vi "Read Response.vi"(8 "error in":errorcluster, 11 "Axis in":refnum<class "Axis.lvclass">) -> (0 "error out":errorcluster, 2 "Success?":bool, 3 "Axis out":refnum<class "Axis.lvclass">)   [LabVIEW 2018, in "Axis.lvlib" / "Axis.lvclass"]
doc: "This VI is used in conjunction with Send Command. Send Command, when using certain types, will send a command to the instrument. Read Response will read the response to make sure the command was valid. Success will be true if the last command was valid."
uses:
  Axis.lvclass
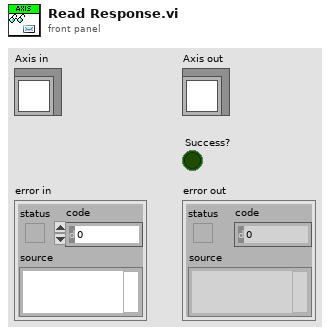
[diagram p1: front panel]
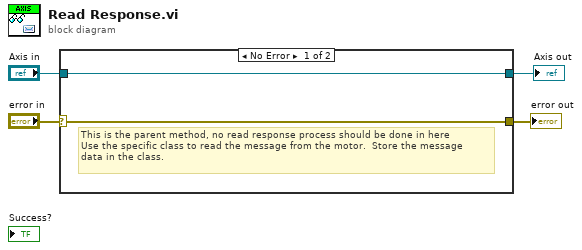
[diagram p0: block diagram]
diagram:
  n1 = case shown="No Error" "error in" {
    selector: "error in" -> [w5 w8]
    tunnel: [w5 w8] -> w3
    tunnel: [w6 w7] -> w1
    tunnel: "Axis in" -> [w6 w7]
    frame No Error {
      # "This is the parent method, no read response process should be done in here\nUse the specific class to read the message from the motor.  Store the message \ndata in the class."
    }
    frame Error {
    }
  }
  "error out" <- w3
  "Axis out" <- w1
